vi "ApplyCLKdialog_2.vi"(10 "CtlRef":refnum<vi>) -> (0 "drop?":bool, 1 "时间（分钟） 2":u32, 2 "时钟出 2":string(combo), 3 "时钟进":string(combo))   [LabVIEW 2015]
panel:
  in  "Cancel":bool
  in  "OK":bool
  in  "时间（分钟）":u32=90
  in  "时钟出":string(combo)="OUT1"
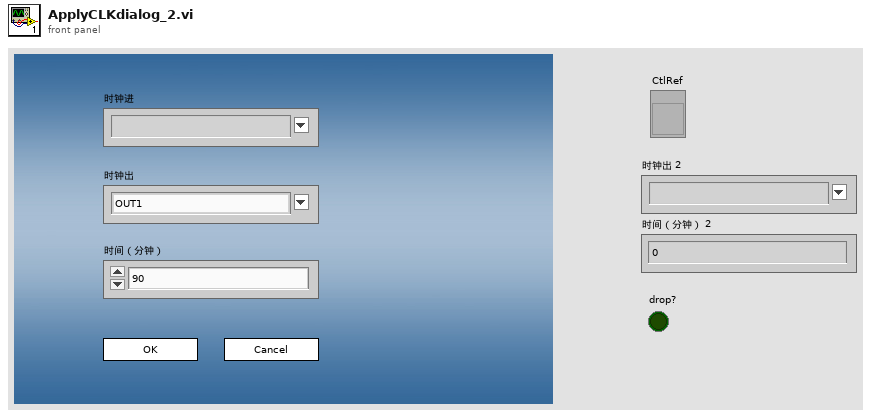
[diagram p1: front panel]
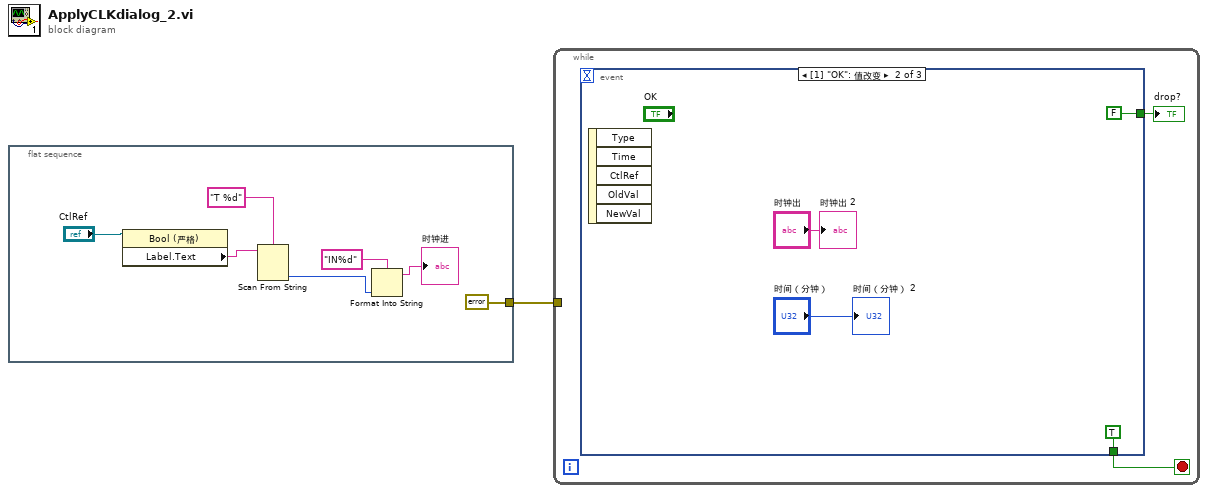
[diagram p0: block diagram]
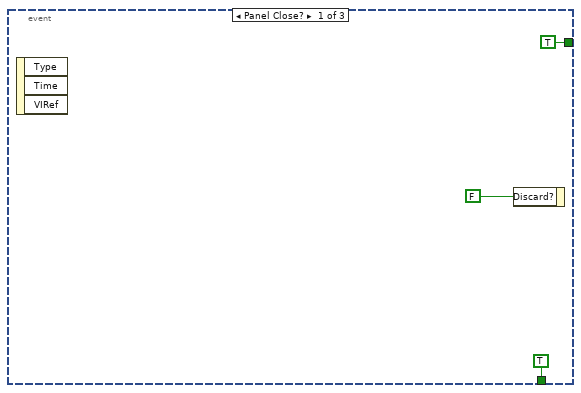
[diagram p2: hidden frame]
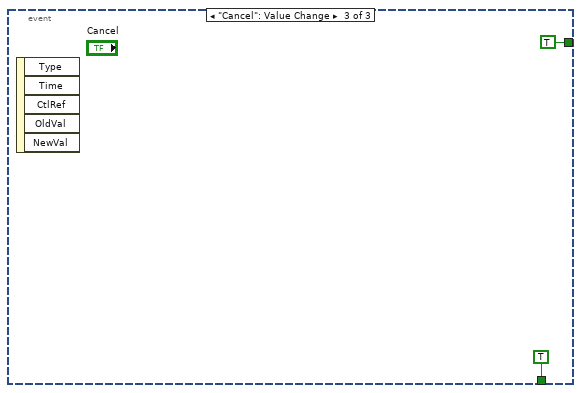
[diagram p3: hidden frame]
diagram:
  n1 = flat-sequence {
    tunnel: [errorcluster {"status"=FALSE, "code"=0, "source"=""} ("error constant")] -> w1
    frame #0 {
      n2 = property class="Bool (严格)"(reference="CtlRef") -> ("Label.Text"=w6:string)  [unwired: 1 in, 2 out]
      n3 = Scan From String(format string="T %d", input string=w6) -> (output 1=w4:i32)  [unwired: 3 in, 3 out]
      n4 = Format Into String(format string="IN%d", w4) -> (resulting string=→"时钟进":string)  [unwired: 2 in, 1 out]
    }
  }
  n5 = while {
    tunnel: w1 -> [_]
    stop <- w9 stop-if-true
    n6 = event shown="[1] \"OK\": 值改变" {
      selector: _ -> [_ _ _]
      dyn-events: _ -> [_ _ _]
      timeout: _ -> [_ _ _]
      tunnel: [TRUE FALSE TRUE] -> w10
      tunnel: [TRUE TRUE TRUE] -> w9
      event Panel Close? {
        n7 = event-data() -> ()  [unwired: 1 in, 3 out]
        n8 = event-data("Discard?"=FALSE ("放弃？")) -> ()  [unwired: 1 in, 1 out]
      }
      event "OK": Value Change {
        n9 = event-data() -> ()  [unwired: 1 in, 5 out]
        "时钟出 2" <- "时钟出"
        "时间（分钟） 2" <- "时间（分钟）"
      }
      event "Cancel": Value Change {
        n10 = event-data() -> ()  [unwired: 1 in, 5 out]
      }
    }
    "drop?" <- w10
  }
